vi "LaunchErrorLogger.vi"(8 "error in (no error)":errorcluster, 11 "TCP_Server in":refnum<class "TCP_Server.lvclass">) -> (0 "error out":errorcluster, 3 "TCP_Server out":refnum<class "TCP_Server.lvclass">)   [LabVIEW 2023, in "TCP_Server.lvlib" / "TCP_Server.lvclass"]
uses:
  TCP_Server.lvclass
  C:/Program Files (x86)/National Instruments/LabVIEW 2023/vi.lib/ActorFramework/Actor/Actor.lvclass
  SimpleErrorLogger/SimpleErrorLogger/SimpleErrorLogger.lvclass
  TCP_Server.lvclass/TCP_Server.ctl
  SimpleErrorLogger/SimpleErrorLogger Messages/Write folder Msg/Write folder Msg.lvclass/Write folder Msg.ctl
  <vilib>/ActorFramework/Message Enqueuer/Message Enqueuer.lvclass/Message Enqueuer.ctl
  SimpleErrorLogger/SimpleErrorLogger Messages/Write filename Msg/Write filename Msg.lvclass/Write filename Msg.ctl
  <vilib>/ActorFramework/Message Enqueuer/Enqueue.vi
  SimpleErrorLogger/SimpleErrorLogger Messages/Write folder Msg/Write folder Msg.lvclass
  C:/Program Files (x86)/National Instruments/LabVIEW 2023/vi.lib/ActorFramework/Message/Message.lvclass
  SimpleErrorLogger/SimpleErrorLogger Messages/Write filename Msg/Write filename Msg.lvclass
  <vilib>/ActorFramework/Message Priority Queue/Priority Enqueue.vi
  <vilib>/ActorFramework/Actor/Actor.lvclass
  SimpleErrorLogger/SimpleErrorLogger Messages/Open Msg/Open Msg.lvclass
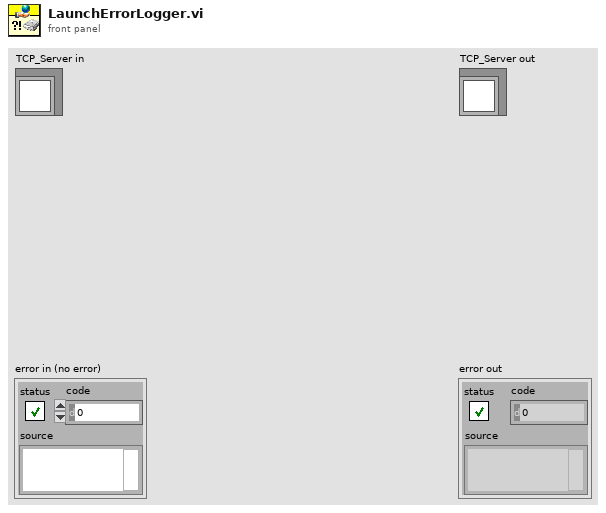
[diagram p1: front panel]
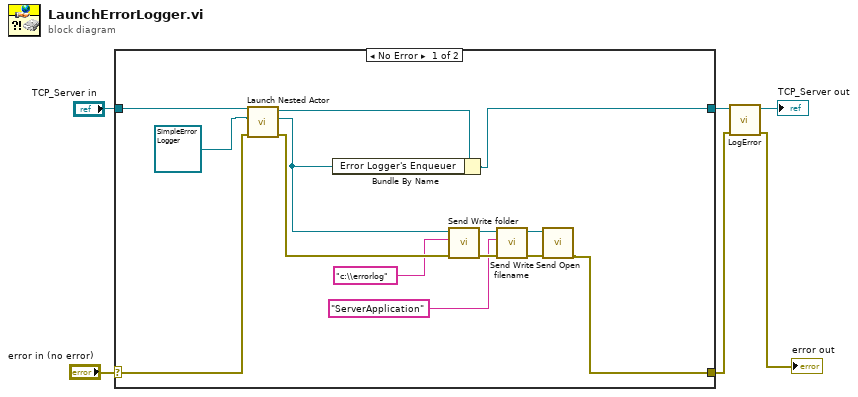
[diagram p0: block diagram]
diagram:
  n1 = case shown="No Error" "error in (no error)" {
    selector: "error in (no error)" -> [w16 w22]
    tunnel: [w7 w22] -> w2
    tunnel: [w17 w21] -> w4
    tunnel: "TCP_Server in" -> [w20 w21]
    frame No Error {
      n2 = call <vilib>:"Launch Nested Actor.vi"("error in (no error)"=w16, "Nested Actor"=refnum<class "SimpleErrorLogger.lvclass"> refnum ("SimpleErrorLogger.lvlib:SimpleErrorLogger.lvclass"), "Caller Actor in"=w20) -> ("error out"=w13:errorcluster, "Nested Actor's Enqueuer"=w15:refnum<class "Message Enqueuer.lvclass">, "Caller Actor out"=w18:refnum<class "TCP_Server.lvclass">)  [unwired: 6 in]
      n3 = Bundle By Name(cluster=w18, "Error Logger's Enqueuer"=w15) -> (w17:refnum<class "TCP_Server.lvclass">)
      n4 = call "Send Write folder.vi"("error in (no error)"=w13, "folder"="c:\\errorlog", "Message Enqueuer"=w15) -> ("error out"=w12:errorcluster, "Message Enqueuer out"=w14:refnum<class "Message Enqueuer.lvclass">)  [unwired: 7 in]
      n5 = call "Send Write filename.vi"("error in (no error)"=w12, "filename"="ServerApplication", "Message Enqueuer"=w14) -> ("error out"=w8:errorcluster, "Message Enqueuer out"=w9:refnum<class "Message Enqueuer.lvclass">)  [unwired: 7 in]
      n6 = call "Send Open.vi"("error in (no error)"=w8, "Message Enqueuer"=w9) -> ("error out"=w7:errorcluster)  [unwired: 8 in, 1 out]
    }
    frame Error {
    }
  }
  n7 = call "LogError.vi"("error in (no error)"=w2, "TCP_Server in"=w4) -> ("error out"=→"error out":errorcluster, "TCP_Server out"=→"TCP_Server out":refnum<class "TCP_Server.lvclass">)  [unwired: 8 in]
